vi "GetAngleByUS.vi"(1 "distance between US":dbl, 3 "d2":dbl, 4 "d1":dbl) -> (0 "alpha":dbl)   [LabVIEW 2016]
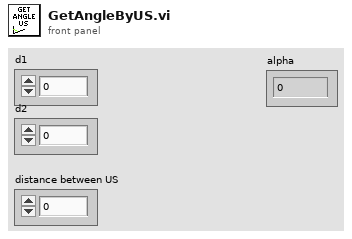
[diagram p1: front panel]
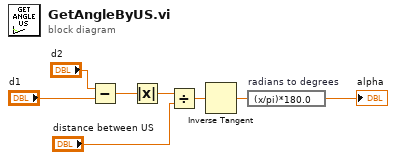
[diagram p0: block diagram]
diagram:
  n1 = Subtract(x="d2", y="d1") -> (x-y=w6:dbl)
  n2 = Absolute Value(x=w6) -> (abs(x)=w5:dbl)
  n3 = Divide(x=w5, y="distance between US") -> (x/y=w3:dbl)
  n4 = Inverse Tangent(1:w3) -> (0:w2:dbl)
  n5 = expression code="(x/pi)*180.0" "radians to degrees"(w2) -> (→"alpha":dbl)
